vi "Discovery Client Resolve Service.vi"(5 "Request Data":T1={"provided_interface"="UnitTestProvidedInterface", "service_class"=""}, 11 "error in (no error)":errorcluster) -> (6 "Response Data":T2, 15 "error out":errorcluster)   [LabVIEW 2020]
uses:
  Discovery Client_lv/Discovery_client/RPC Messages/ni_measurementlink_discovery_v1_ServiceLocation.ctl
  Discovery Client_lv/Discovery_client/RPC Messages/ni_measurementlink_discovery_v1_ResolveServiceRequest.ctl
  Discovery Client_lv/Discovery_client/Discovery_client.lvlib
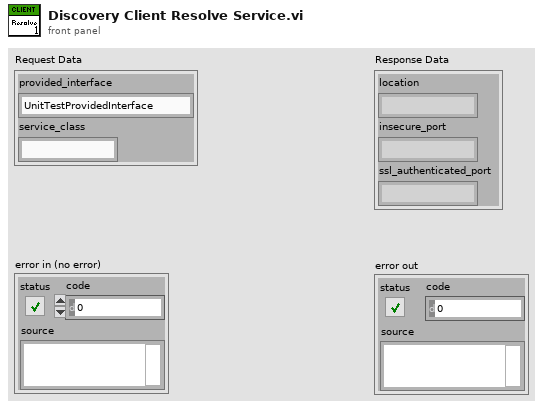
[diagram p1: front panel]
types:
  T1 = typedef "Discovery_client.lvlib/ni_measurementlink_discovery_v1_ResolveServiceRequest.ctl" = cluster{"provided_interface":string, "service_class":string}
  T2 = typedef "Discovery_client.lvlib/ni_measurementlink_discovery_v1_ServiceLocation.ctl" = cluster{"location":string, "insecure_port":string, "ssl_authenticated_port":string}
  T3 = typedef "grpc-lvsupport-release.lvlib/grpcId.ctl" = u64
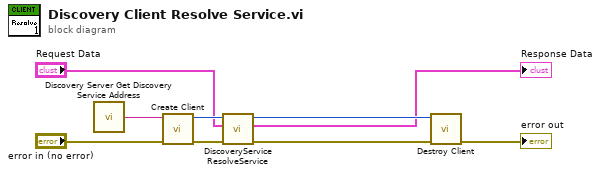
[diagram p0: block diagram]
diagram:
  n1 = call "Discovery Server Get Discovery Service Address.vi"() -> ("address"=w9:string)  [unwired: 15 in]
  n2 = call "Create Client.vi"("error in"="error in (no error)", "address"=w9) -> ("error out"=w7:errorcluster, "gRPC ID Out"=w6:T3)  [unwired: 8 in]
  n3 = call "DiscoveryService ResolveService.vi"("error in"=w7, "Request Data"="Request Data", "gRPC ID"=w6) -> ("error out"=w5:errorcluster, "Response Data"=→"Response Data":T2, "gRPC ID out"=w4:T3)  [unwired: 6 in]
  n4 = call "Destroy Client.vi"("error in"=w5, "gRPC ID"=w4) -> ("error out"=→"error out":errorcluster)  [unwired: 9 in]
